vi "Result_Test.vi"(8 "error in (no error)":errorcluster caption="entrée d'erreur (pas d'erreur)", 11 "Get_Voltage en entrée":refnum<class "Nodon_Start_ZCR.lvclass">) -> (0 "error out":errorcluster caption="sortie d'erreur", 3 "Get_Voltage en sortie":refnum<class "Nodon_Start_ZCR.lvclass">)   [LabVIEW 2020, in "Library Test.lvlib" / "Nodon_Start_ZCR.lvclass"]
uses:
  Nodon_Start_ZCR.lvclass
  C:/Users/ngarcin/OneDrive - Altyor/Standard TB/Suite TB45/Class/Test/Test (Default)/Test (Default).lvclass
  Commun VI/TypeDef/Variable Printable.ctl
  JSON API/JSON Value/Set from JSON string.vi
  JSON API/JSON Value/JSON Value.lvclass
  Nodon_Send_Command_UART/Nodon_Send_Command_UART.lvclass
  JSON API/Variant JSON/Variant JSON.lvlib
  JSON API/Get Polymorphic/JSON GetSet.lvlib
  Commun VI/Library Commun.lvlib
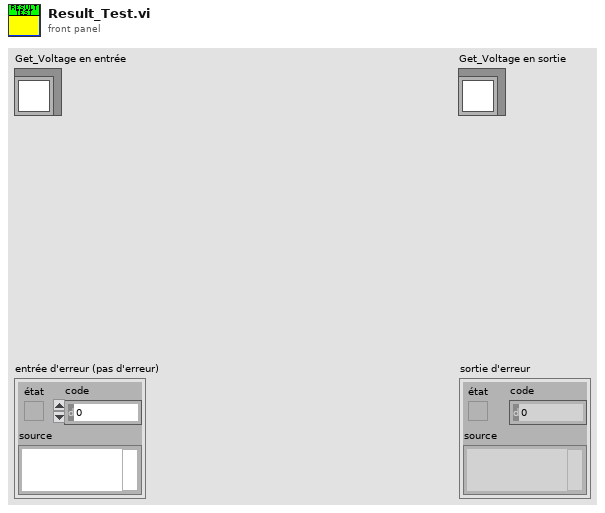
[diagram p1: front panel]
types:
  T1 = typedef "Variable Printable.ctl" = string
  T2 = enum16{"Get Variable", "Get All Variables", "Set Variable", "Delete Variable", "Delete All Variable"}
  T3 = cluster{"Commande Type":string, "Command ID":string, "Data":string, "Error":string}
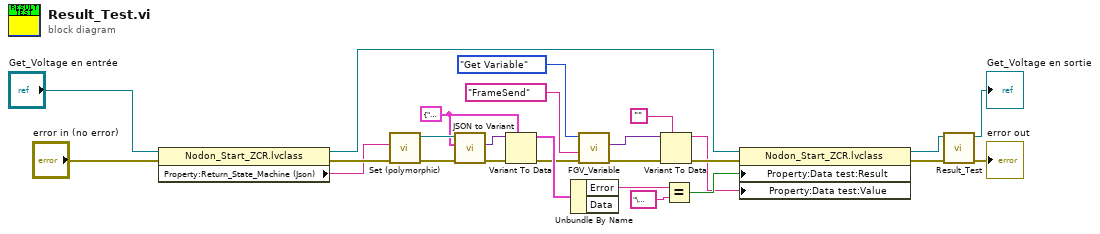
[diagram p0: block diagram]
diagram:
  w13 = T3 {"Commande Type"="", "Command ID"="", "Data"="", "Error"=""}
  n1 = property class="Nodon_Start_ZCR.lvclass"(reference="Get_Voltage en entrée", error in="error in (no error)") -> (reference out=w24:refnum<class "Nodon_Start_ZCR.lvclass">, error out=w19:errorcluster, "Property:Return_State_Machine (Json)"=w18:string)
  n2 = call-poly "Set (polymorphic).vi"("error in (no error)"=w19, "JSON stream"=w18) -> ("error out"=w21:errorcluster, "JSON Value out"=w23:refnum<class "JSON Value.lvclass">)  [unwired: 7 in, 1 out]
  n3 = call "JSON to Variant.vi"("error in (no error)"=w21, "Variant (Data Type)"=w13, "JSON Value"=w23) -> ("error out"=w22:errorcluster, "Variant out"=w20:variant)  [unwired: 7 in]
  n4 = Variant To Data(error in=w22, type=w13, Variant=w20) -> (data=w17:T3, error out=w3:errorcluster)
  n5 = Unbundle By Name(w17) -> ("Error"=w16:string)  [unwired: 1 out]
  n6 = call "FGV_Variable.vi"("error in (no error)"=w3, "Variable"=T1 "FrameSend", "Function"=T2."Get Variable") -> ("error out"=w5:errorcluster, "Data Out"=w6:variant)  [unwired: 6 in, 1 out]
  n7 = Variant To Data(error in=w5, type="", Variant=w6) -> (data=w1:string, error out=w2:errorcluster)
  n8 = Equal?(x=w16, y="\u0000") -> (x = y?=w14:bool)
  n9 = property class="Nodon_Start_ZCR.lvclass"(reference=w24, error in=w2, "Property:Data test:Result"=w14, "Property:Data test:Value"=w1) -> (reference out=w10:refnum<class "Nodon_Start_ZCR.lvclass">, error out=w9:errorcluster)
  n10 = call-parent "Result_Test.vi"("error in (no error)"=w9, "Get_Voltage en entrée"=w10) -> ("error out"=→"error out":errorcluster, "Get_Voltage en sortie"=→"Get_Voltage en sortie":refnum<class "Nodon_Start_ZCR.lvclass">)  [unwired: 8 in]
